vi "startSweepAndWait.vi"(8 "error in (no error)":errorcluster, 10 "SweepConfiguration":T3, 11 "Instrument.Lockin in":refnum<class "Instrument.Lockin.lvclass">) -> (0 "error out":errorcluster, 1 "Results":T1, 2 "Waveforms":T2, 3 "Instrument.Lockin out":refnum<class "Instrument.Lockin.lvclass">)   [LabVIEW 2019, in "Instrument.Lockin.lvclass"]
uses:
  Instrument.Lockin.lvclass
  <userlib>/LevyLab/Instrument Framework/Instrument Types/Lockin/Instrument.LockinAPI.lvclass
  <userlib>/LevyLab/Instrument Framework/Instrument Types/Lockin/Typedefs/LockinAPI.SweepChannel--Cluster.ctl
  <userlib>/LevyLab/Instrument Framework/Instrument Types/Lockin/Typedefs/LockinAPI.SweepConfig--Cluster.ctl
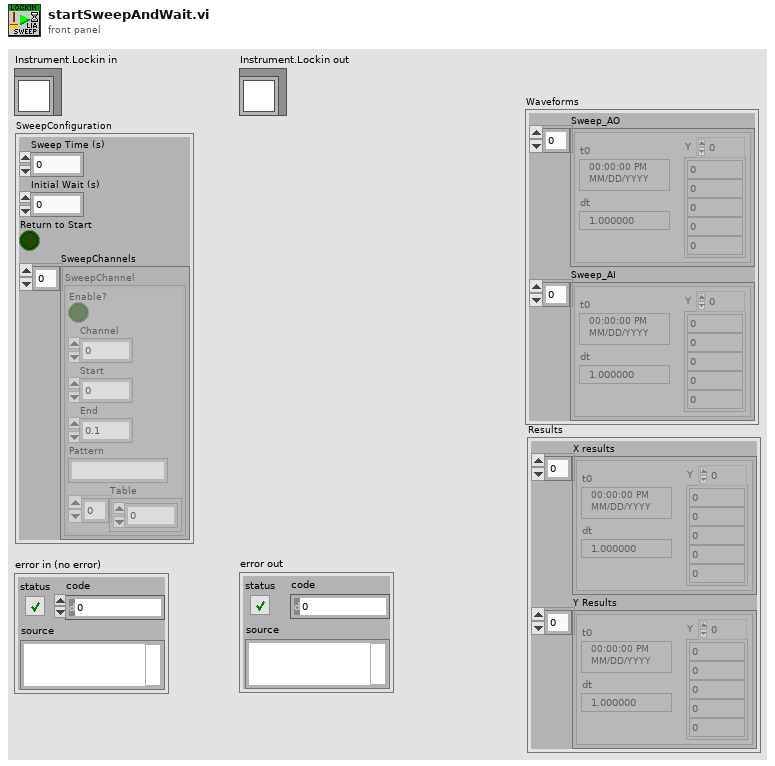
[diagram p1: front panel]
types:
  T1 = cluster{"X results":waveform(dbl)[], "Y Results":waveform(dbl)[]}
  T2 = cluster{"Sweep_AO":waveform(dbl)[], "Sweep_AI":waveform(dbl)[]}
  T3 = typedef "Instrument.LockinAPI.lvclass/LockinAPI.SweepConfig--Cluster.ctl" = cluster{"Sweep Time (s)":dbl, "Initial Wait (s)":dbl, "Return to Start":bool, "SweepChannels":T4[]}
  T4 = typedef "Instrument.LockinAPI.lvclass/LockinAPI.SweepChannel--Cluster.ctl" = cluster{"Enable?":bool, "Channel":u16, "Start":dbl, "End":dbl, "Pattern":string, "Table":dbl[]}
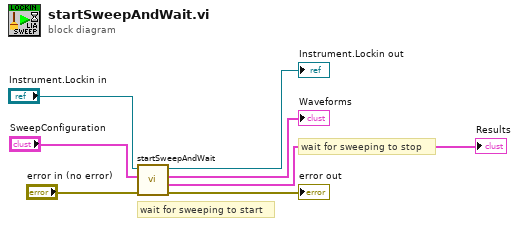
[diagram p0: block diagram]
diagram:
  # "wait for sweeping to stop"
  # "wait for sweeping to start"
  n1 = call-parent "startSweepAndWait.vi"("error in (no error)"="error in (no error)", "SweepConfiguration"="SweepConfiguration", "Instrument.LockinAPI in"="Instrument.Lockin in") -> ("error out"=→"error out":errorcluster, "Results"=→"Results":T1, "Waveforms"=→"Waveforms":T2, "Instrument.LockinAPI out"=→"Instrument.Lockin out":refnum<class "Instrument.Lockin.lvclass">)  [unwired: 5 in]
